vi "Create data array.vi"(4 "error in":errorcluster, 5 "input main cluster":T2, 7 "Map geometry":T1) -> (0 "error out":errorcluster, 1 "output main cluster":T2, 2 "Data array":dbl[][](array[numeric]), 3 "Map geometry out":T1)   [LabVIEW 2010]
uses:
  Main_cluster.ctl
  <vilib>/vision/Image Controls.llb/IMAQ Image.ctl
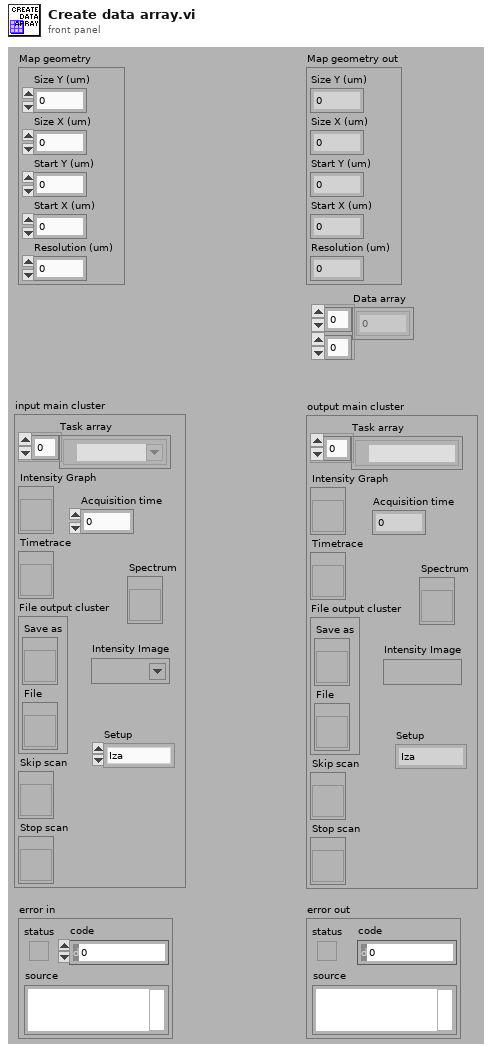
[diagram p1: front panel]
types:
  T1 = cluster{"Size Y (um)":dbl, "Size X (um)":dbl, "Start Y (um)":dbl, "Start X (um)":dbl, "Resolution (um)":dbl}
  T2 = typedef "Main_cluster.ctl" = cluster{"Task array":refnum<k21>[], "Intensity Graph":refnum<vi>, "Timetrace":refnum<vi>, "File output cluster":cluster{"Save as":refnum<vi>, "File":refnum<vi>}, "Skip scan":refnum<vi>, "Stop scan":refnum<vi>, "Acquisition time":dbl, "Setup":enum16{"Iza", "Lukasz"}, "Spectrum":refnum<vi>, "Intensity Image":T3}
  T3 = typedef "IMAQ Image.ctl" = refnum<image>
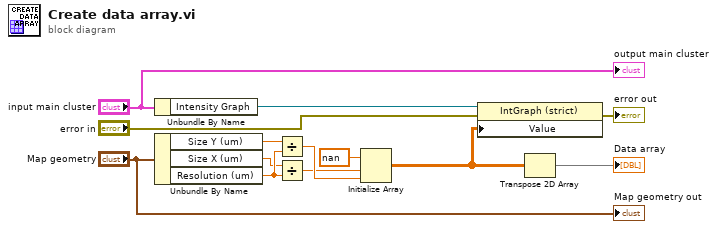
[diagram p0: block diagram]
diagram:
  n1 = Unbundle By Name("input main cluster") -> ("Intensity Graph"=w11:refnum<vi>)
  n2 = Unbundle By Name("Map geometry") -> ("Size Y (um)"=w3:dbl, "Size X (um)"=w4:dbl, "Resolution (um)"=w5:dbl)
  n3 = Divide(x=w3, y=w5) -> (x/y=w8:dbl)
  n4 = Divide(x=w4, y=w5) -> (x/y=w7:dbl)
  n5 = Initialize Array(nan ("Numeric"), w7, w8) -> (w6:dbl[][])
  n6 = property class="IntGraph (strict)"(reference=w11, error in="error in", "Value"=w6) -> (error out=→"error out":errorcluster)  [unwired: 1 out]
  n7 = Transpose 2D Array(2D array=w6) -> (transposed array=→"Data array":dbl[][])
  "output main cluster" <- "input main cluster"
  "Map geometry out" <- "Map geometry"
